vi "Test View Broadcast When View is Hidden.vi"(8 "error in (no error)":errorcluster, 11 "UI View Test In":refnum<class "View Test.lvclass">) -> (0 "error out":errorcluster, 3 "UI View Test Out":refnum<class "View Test.lvclass">)   [LabVIEW 2020, in "View Test.lvclass"]
uses:
  View Test.lvclass
  C:/Program Files (x86)/National Instruments/LabVIEW 2020/vi.lib/Asteme/LUnit/Test Case.lvclass
  Framework/Process/Process.lvclass/Process.ctl
  Framework/View/View.lvclass/View.ctl
  <vilib>/Asteme/LUnit/Test Case.lvclass/Test Case.ctl
  <vilib>/Asteme/LUnit/LUnit Assertion Result.lvclass/LUnit Assertion Result.ctl
  Framework/Broadcast Event Helpers/Execution timer.vi
  Framework/Process/Protected/Messaging/Enqueue Message.vi
  Framework/View/Public/Get View VI Reference.vi
  <vilib>/Utility/error.llb/Clear Errors.vi
  Framework/Process/Public/Lifecycle/Get Lifecycle State.vi
  Framework/Process/Private/SubVIs/Wait for finish.vi
  Framework/Process/Private/SubVIs/Set Lifecycle State.vi
  <vilib>/Asteme/LUnit/Palette/Pass.vi
  <vilib>/Asteme/LUnit/Palette/Fail.vi
  <vilib>/Asteme/LUnit/Variant to string.vi
  <vilib>/Asteme/LUnit/Set Assertion Type.vi
  Framework/Process/Protected/Messaging/Request Message.vi
  <vilib>/Asteme/LUnit/Add test result.vi
  <vilib>/Asteme/LUnit/LUnit Write Passed.vi
  <vilib>/Asteme/LUnit/LUnit Get Test Case.vi
  <vilib>/Asteme/LUnit/Assertion Result/LUnit Get Test Name.vi
  <vilib>/Asteme/LUnit/LUnit Write Message.vi
  <vilib>/Asteme/LUnit/LUnit Write Description.vi
  <vilib>/Asteme/LUnit/LUnit Write Assertion Type.vi
  Framework/Process/Private/SubVIs/Enqueue Request Message.vi
  <vilib>/Asteme/LUnit/Read Test Case Name.vi
  Framework/View/View.lvclass
  C:/Users/anton/Documents/GitHub/Triarc-Framework/source/Framework/Process/Process.lvclass
  <vilib>/Utility/error.llb/Error Cluster From Error Code.vi
  Framework/Process/Private/SubVIs/Wait for Response Message.vi
  Framework/Broadcast Event Helpers/Dequeue Broadcast Message.vi
  <vilib>/Utility/Data Type/Get Type Information.vi
  <vilib>/Utility/LVClass/Get LV Class Name.vi
  <vilib>/Asteme/LUnit/LUnit Assertion Result.lvclass
  Framework/Process/Process.lvclass
  Framework/Broadcast Event Helpers/Broadcast Event Helpers.lvlib
  <vilib>/Asteme/LUnit/Test Case.lvclass
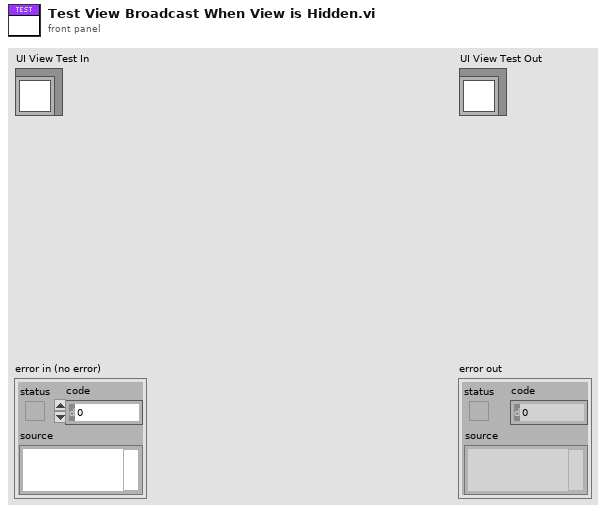
[diagram p1: front panel]
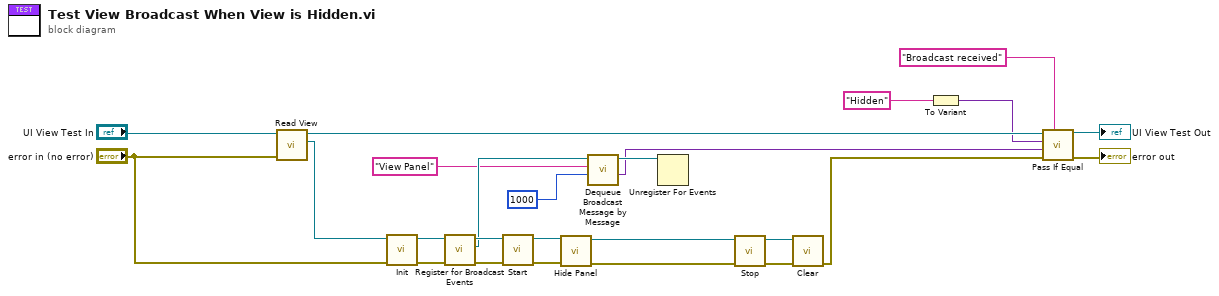
[diagram p0: block diagram]
diagram:
  n1 = call "Read View.vi"("error in (no error)"="error in (no error)", "View Test In"="UI View Test In") -> ("View"=w20:refnum<class "View.lvclass">, "View Test Out"=w23:refnum<class "View Test.lvclass">)  [unwired: 7 in, 1 out]
  n2 = call-dynamic "Init.vi"("error in (no error)"="error in (no error)", "View In"=w20) -> ("error out"=w15:errorcluster, "View Out"=w10:refnum<class "View.lvclass">)  [unwired: 8 in]
  n3 = call "Register for Broadcast Events.vi"("error in (no error)"=w15, "Process In"=w10) -> ("error out"=w11:errorcluster, "Event Registration Refnum Out"=w8:refnum<event-registration>, "Process Out"=w9:refnum<class "View.lvclass">)  [unwired: 7 in]
  n4 = call "Start.vi"("error in (no error)"=w11, "Process In"=w9) -> ("error out"=w18:errorcluster, "Process Out"=w19:refnum<class "View.lvclass">)  [unwired: 8 in]
  n5 = call "Hide Panel.vi"("error in (no error)"=w18, "View In"=w19) -> ("error out"=w12:errorcluster, "View Out"=w13:refnum<class "View.lvclass">)  [unwired: 8 in]
  n6 = call "Dequeue Broadcast Message by Message.vi"("Timeout (-1)"=1000, "Message"="View Panel", "Event Registration Refnum"=w8) -> ("Message Data"=w3:variant, "Event Registration Refnum Out"=w5:refnum<event-registration>)  [unwired: 4 in, 3 out]
  n7 = Unregister For Events(event registration refnum=w5) -> ()  [unwired: 1 in, 1 out]
  n8 = call "Stop.vi"("error in (no error)"=w12, "Process In"=w13) -> ("error out"=w16:errorcluster, "Process Out"=w17:refnum<class "View.lvclass">)  [unwired: 7 in, 1 out]
  n9 = call-dynamic "Clear.vi"("error in (no error)"=w16, "View In"=w17) -> ("error out"=w4:errorcluster)  [unwired: 9 in]
  n10 = To Variant(anything="Hidden") -> (Variant=w1:variant)
  n11 = call <vilib>:"Pass If Equal.vi"("Description"="Broadcast received", "error in (no error)"=w4, "Actual"=w3, "Expected"=w1, "Test Case In"=w23) -> ("error out"=→"error out":errorcluster, "Test Case Out"=→"UI View Test Out":refnum<class "View Test.lvclass">)  [unwired: 5 in]
